vi "copy.vi"(8 "error in (no error)":errorcluster, 10 "image to copy (source)":refnum<class "Image.lvclass">, 11 "Image in (target)":refnum<class "Image.lvclass">) -> (0 "error out":errorcluster, 3 "Image out":refnum<class "Image.lvclass">)   [LabVIEW 2010, in "Image.lvclass"]
uses:
  Image.lvclass
  Image.lvclass/Image.ctl
  ErrorController/ErrorController/class_data.vi
  ErrorController/ErrorController/ErrorController.lvclass
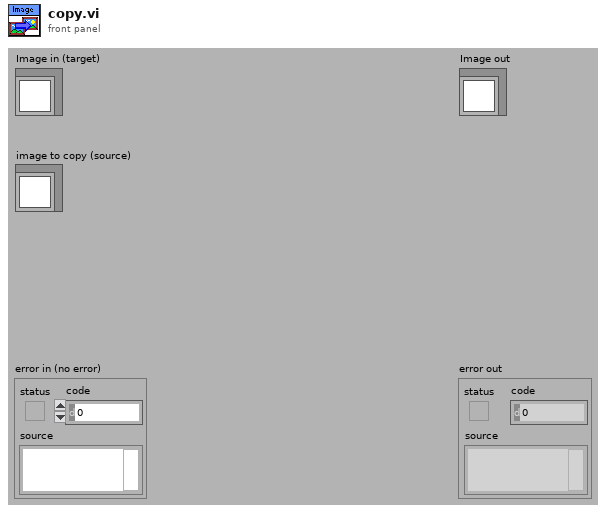
[diagram p1: front panel]
types:
  T1 = typedef "Image.lvclass/unit.ctl" = enum16{"um", "s"}
  T2 = typedef "Image.lvclass/storage_mode.ctl" = enum16{"RAM", "disk"}
  T3 = typedef "IMAQ Image.ctl" = refnum<image>
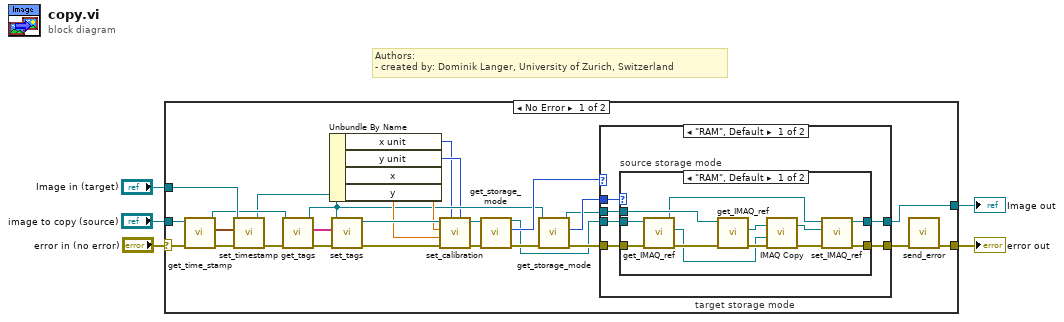
[diagram p0: block diagram]
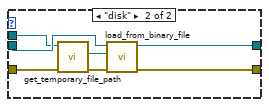
[diagram p2: hidden frame]
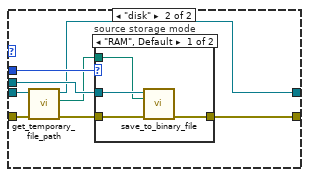
[diagram p3: hidden frame]
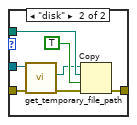
[diagram p4: hidden frame]
diagram:
  # "Authors: \n- created by: Dominik Langer, University of Zurich, Switzerland"
  n1 = case shown="No Error" "error in (no error)" {
    selector: "error in (no error)" -> [w28 w79]
    tunnel: [w7 w79] -> w4
    tunnel: [w29 w78] -> w2
    tunnel: "Image in (target)" -> [w25 w78]
    tunnel: "image to copy (source)" -> [w27 _]
    frame No Error {
      n2 = call-dynamic "get_time_stamp.vi"("error in (no error)"=w28, "Image.lvclass in"=w27) -> ("error out"=w26:errorcluster, "timestamp"=w24:timestamp, "Image.lvclass out"=w20:refnum<class "Image.lvclass">)  [unwired: 7 out]
      n3 = call-dynamic "set_timestamp.vi"("error in (no error)"=w26, "timestamp"=w24, "Image.lvclass in"=w25) -> ("error out"=w23:errorcluster, "Image.lvclass out"=w19:refnum<class "Image.lvclass">)  [unwired: 7 out]
      n4 = call "get_tags.vi"("error in (no error)"=w23, "Image.lvclass in"=w20) -> ("error out"=w22:errorcluster, "tags"=w21:string[], "Image.lvclass out"=w11:refnum<class "Image.lvclass">)  [unwired: 7 out]
      n5 = Unbundle By Name(w11) -> ("x unit"=w8:T1, "y unit"=w9:T1, "x"=w14:dbl, "y"=w13:dbl)
      n6 = call "set_tags.vi"("error in (no error)"=w22, "tags"=w21, "Image.lvclass in"=w19) -> ("error out"=w15:errorcluster, "Image.lvclass out"=w18:refnum<class "Image.lvclass">)  [unwired: 7 out]
      n7 = call "set_calibration.vi"("y unit"=w9, "x unit"=w8, "error in (no error)"=w15, "y"=w13, "x"=w14, "Image in"=w18) -> ("error out"=w17:errorcluster, "Image out"=w16:refnum<class "Image.lvclass">)  [unwired: 4 out]
      n8 = call-dynamic "get_storage_mode.vi"("error in (no error)"=w17, "Image.lvclass in"=w16) -> ("error out"=w33:errorcluster, "storage mode"=w31:T2, "Image.lvclass out"=w12:refnum<class "Image.lvclass">)  [unwired: 7 out]
      n9 = call-dynamic "get_storage_mode.vi"("error in (no error)"=w33, "Image.lvclass in"=w11) -> ("error out"=w32:errorcluster, "storage mode"=w30:T2, "Image.lvclass out"=w10:refnum<class "Image.lvclass">)  [unwired: 7 out]
      n10 = case "target storage mode" shown="\"RAM\", Default" w31 {
        tunnel: [w38 w66] -> w6
        tunnel: w32 -> [w39 w63]
        tunnel: w30 -> [w37 w65]
        tunnel: w10 -> [w34 w64]
        tunnel: w12 -> [w36 w61]
        tunnel: [w35 w59] -> w29
        frame "RAM", Default {
          n11 = case "source storage mode" shown="\"RAM\", Default" w37 {
            tunnel: [w43 w58] -> w38
            tunnel: w39 -> [w48 w56]
            tunnel: w36 -> [w51 w54]
            tunnel: [w41 w57] -> w35
            tunnel: w34 -> [w50 w53]
            frame "RAM", Default {
              n12 = call-dynamic "get_IMAQ_ref.vi"("error in (no error)"=w48, "Image.lvclass in"=w51) -> ("error out"=w49:errorcluster, "Image"=w45:T3, "Image.lvclass out"=w42:refnum<class "Image.lvclass">)  [unwired: 7 out]
              n13 = call-dynamic "get_IMAQ_ref.vi"("error in (no error)"=w49, "Image.lvclass in"=w50) -> ("error out"=w47:errorcluster, "Image"=w46:T3)  [unwired: 8 out]
              n14 = call "IMAQ Copy"("error in (no error)"=w47, "Image Dst"=w45, "Image Src"=w46) -> ("error out"=w44:errorcluster, "Image Dst Out"=w40:T3)  [unwired: 3 out]
              n15 = call-dynamic "set_IMAQ_ref.vi"("error in (no error)"=w44, "Image"=w40, "Image.lvclass in"=w42) -> ("error out"=w43:errorcluster, "Image.lvclass out"=w41:refnum<class "Image.lvclass">)  [unwired: 7 out]
            }
            frame "disk" {
              n16 = call-dynamic "get_temporary_file_path.vi"("error in (no error)"=w56, "Image.lvclass in"=w53) -> ("error out"=w55:errorcluster, "temporary file path"=w52:path)  [unwired: 8 out]
              n17 = call-dynamic "load_from_binary_file.vi"("error in (no error)"=w55, "Path"=w52, "Image in"=w54) -> ("error out"=w58:errorcluster, "Image out"=w57:refnum<class "Image.lvclass">)  [unwired: 7 out]
            }
          }
        }
        frame "disk" {
          n18 = call-dynamic "get_temporary_file_path.vi"("error in (no error)"=w63, "Image.lvclass in"=w61) -> ("error out"=w62:errorcluster, "temporary file path"=w60:path, "Image.lvclass out"=w59:refnum<class "Image.lvclass">)  [unwired: 7 out]
          n19 = case "source storage mode" shown="\"RAM\", Default" w65 {
            tunnel: [w70 w77] -> w66
            tunnel: w62 -> [w67 w74]
            tunnel: w64 -> [w69 w72]
            tunnel: w60 -> [w68 w76]
            frame "RAM", Default {
              n20 = call-dynamic "save_to_binary_file.vi"("error in (no error)"=w67, "Path"=w68, "Image in"=w69) -> ("error out"=w70:errorcluster)  [unwired: 5 in, 3 out]
            }
            frame "disk" {
              n21 = call-dynamic "get_temporary_file_path.vi"("error in (no error)"=w74, "Image.lvclass in"=w72) -> ("error out"=w73:errorcluster, "temporary file path"=w71:path)  [unwired: 8 out]
              n22 = Copy(8:w73, 9:TRUE ("overwrite (F)"), 10:w76, 11:w71) -> (0:w77:errorcluster)  [unwired: 3 out]
            }
          }
        }
      }
      n23 = call "send_error.vi"("error in (no error)"=w6) -> ("error out"=w7:errorcluster)  [unwired: 10 in]
    }
    frame Error {
    }
  }
  "error out" <- w4
  "Image out" <- w2
